vi "Init - Find Duplex.vi"(8 "error in (no error)":errorcluster, 11 "Compiled.Settings in":T1 {"Tx Packet Info"."targetPriority" min=1 step=1; "Tx Packet Info"."targetProcessor" min=-2 max=16 step=1; "Tx Packet Info"."Endianness" items=["big-endian"=0, "little-indian"=2]; "Rx Packet Info"."Endianness" items=["big-endian"=0, "little-indian"=2]}) -> (0 "error out":errorcluster, 3 "Compiled.Settings out":T1 {"Tx Packet Info"."targetPriority" min=1 step=1; "Tx Packet Info"."targetProcessor" min=-2 max=16 step=1; "Tx Packet Info"."Endianness" items=["big-endian"=0, "little-indian"=2]; "Rx Packet Info"."Endianness" items=["big-endian"=0, "little-indian"=2]})   [LabVIEW 2019, in "UDP-Custom-Device Engine.lvlib"]
uses:
  UDP-Custom-Device Engine.lvlib
  Shared/Compiled.Settings.ctl
  Shared/Types/Shared - Rx.PacketInfo.ctl
  Shared/Types/Shared - Channel Data Type.ctl
  Shared/Types/Shared - Buffered.PacketInfo.ctl
  Shared/Types/Shared - Pointer Encoding.ctl
  Shared/Types/Shared - Receive Buffer Options.ctl
  Shared/Types/Shared - Transmit Buffer Options.ctl
  Shared/Types/Shared - Duplex Settings.ctl
  Shared/Types/Shared - New Data Options.ctl
  Shared/Types/Shared - Thread Management.ctl
  Shared/Types/Shared - Tx.PacketInfo.ctl
  Shared/Types/Shared - Transmit Flag Options.ctl
  Shared/Types/Shared - Transmit Echo Options.ctl
  Shared/Types/Shared - Transmit Sim Options.ctl
  Shared/Types/Shared - Header Details.ctl
  Shared/Types/Shared - Custom Header.ctl
  Shared/UDP-Custom-Device Shared.lvlib
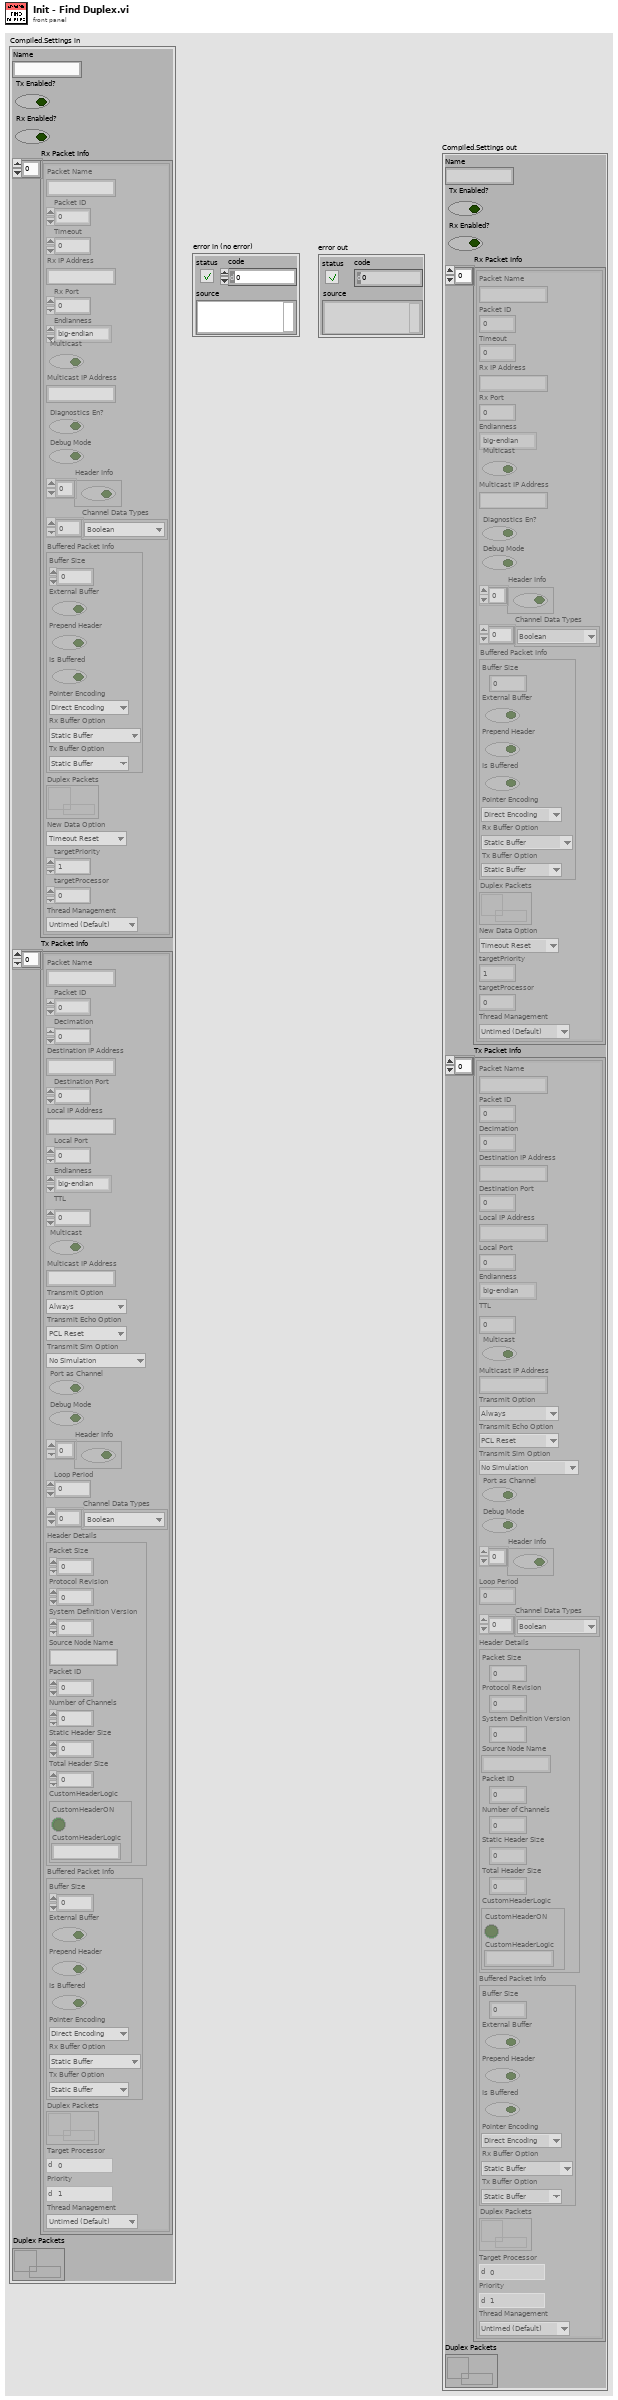
[diagram p1: front panel]
types:
  T1 = typedef "UDP-Custom-Device Shared.lvlib/Compiled.Settings.ctl" = cluster{"Name":string, "Tx Enabled?":bool, "Rx Enabled?":bool, "Rx Packet Info":T2[], "Tx Packet Info":T10[], "Duplex Packets":refnum<data-value>}
  T2 = typedef "UDP-Custom-Device Shared.lvlib/Shared - Rx.PacketInfo.ctl" = cluster{"Packet Name":string, "Packet ID":i32, "Timeout":i32, "Rx IP Address":string, "Rx Port":u16, "Endianness":u16, "Multicast":bool, "Multicast IP Address":string, "Diagnostics En?":bool, "Debug Mode":bool, "Header Info":bool[], "Channel Data Types":T3[], "Buffered Packet Info":T4, "Duplex Packets":refnum<data-value>, "New Data Option":T8, "targetPriority":i16, "targetProcessor":i8, "Thread Management":T9}
  T3 = typedef "UDP-Custom-Device Shared.lvlib/Shared - Channel Data Type.ctl" = enum16{"Boolean", "Single", "Double", "I8", "I16", "I32", "I64", "U8", "U16", "U32", "U64"}
  T4 = typedef "UDP-Custom-Device Shared.lvlib/Shared - Buffered.PacketInfo.ctl" = cluster{"Buffer Size":i32, "External Buffer":bool, "Prepend Header":bool, "Is Buffered":bool, "Pointer Encoding":T5, "Rx Buffer Option":T6, "Tx Buffer Option":T7}
  T5 = typedef "UDP-Custom-Device Shared.lvlib/Shared - Pointer Encoding.ctl" = enum16{"Direct Encoding", "Conversion Encoding"}
  T6 = typedef "UDP-Custom-Device Shared.lvlib/Shared - Receive Buffer Options.ctl" = enum16{"Static Buffer", "Circular Buffer", "Circular Buffer + Size", "Internal Cache", "Internal Cache + Size", "Ping Pong", "Ping Pong + Size"}
  T7 = typedef "UDP-Custom-Device Shared.lvlib/Shared - Transmit Buffer Options.ctl" = enum16{"Static Buffer", "FIFO Buffer", "FIFO Buffer + Port"}
  T8 = typedef "UDP-Custom-Device Shared.lvlib/Shared - New Data Options.ctl" = enum16{"Timeout Reset", "Counter"}
  T9 = typedef "UDP-Custom-Device Shared.lvlib/Shared - Thread Management.ctl" = enum16{"Untimed (Default)", "Timed (High Priority)"}
  T10 = typedef "UDP-Custom-Device Shared.lvlib/Shared - Tx.PacketInfo.ctl" = cluster{"Packet Name":string, "Packet ID":i32, "Decimation":u16, "Destination IP Address":string, "Destination Port":u16, "Local IP Address":string, "Local Port":u16, "Endianness":u16, "TTL":u16, "Multicast":bool, "Multicast IP Address":string, "Transmit Option":T11, "Transmit Echo Option":T12, "Transmit Sim Option":T13, "Port as Channel":bool, "Debug Mode":bool, "Header Info":bool[], "Loop Period":u32, "Channel Data Types":T3[], "Header Details":T14, "Buffered Packet Info":T4, "Duplex Packets":refnum<data-value>, "targetProcessor":i8, "targetPriority":i16, "Thread Management":T9}
  T11 = typedef "UDP-Custom-Device Shared.lvlib/Shared - Transmit Flag Options.ctl" = enum16{"Always", "One-Shot", "Toggle"}
  T12 = typedef "UDP-Custom-Device Shared.lvlib/Shared - Transmit Echo Options.ctl" = enum16{"PCL Reset", "Counter", "Mirror"}
  T13 = typedef "UDP-Custom-Device Shared.lvlib/Shared - Transmit Sim Options.ctl" = enum16{"No Simulation", "Counter", "Full Buffer", "FIFO Test", "FIFO + Port Test"}
  T14 = typedef "UDP-Custom-Device Shared.lvlib/Shared - Header Details.ctl" = cluster{"Packet Size":u16, "Protocol Revision":u8, "System Definition Version":u64, "Source Node Name":string, "Packet ID":u32, "Number of Channels":u32, "Static Header Size":u16, "Total Header Size":u16, "CustomHeaderLogic":T15}
  T15 = typedef "UDP-Custom-Device Shared.lvlib/Shared - Custom Header.ctl" = cluster{"CustomHeaderON":bool, "CustomHeaderLogic":string}
  T16 = typedef "UDP-Custom-Device Shared.lvlib/Shared - Duplex Settings.ctl" = cluster{"Transmit Packet ID":i32, "Receive Packet ID":i32, "Multicast":bool, "Multicast Address":string, "IP Address":string, "Port":u16, "TTL":u16, "Duplex Connection":refnum<k16>}
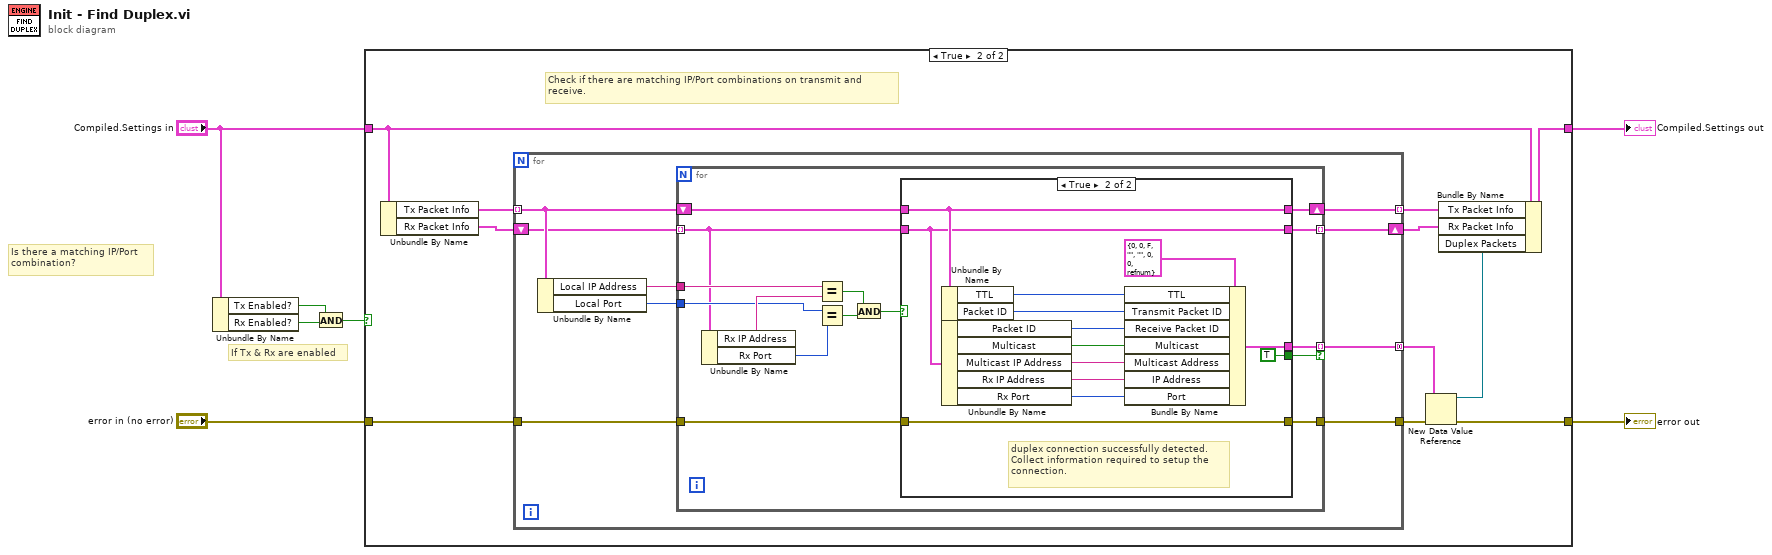
[diagram p0: block diagram]
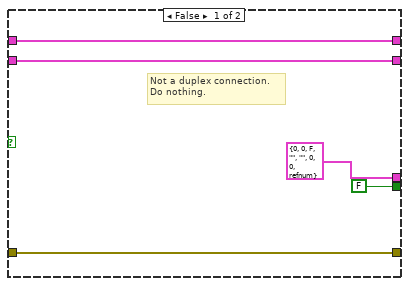
[diagram p3: hidden frame]
diagram:
  # "Is there a matching IP/Port\ncombination?"
  # "If Tx & Rx are enabled"
  n1 = Unbundle By Name("Compiled.Settings in") -> ("Tx Enabled?"=w4:bool, "Rx Enabled?"=w5:bool)
  n2 = And(x=w4, y=w5) -> (x .and. y?=w3:bool)
  n3 = case shown="True" w3 {
    tunnel: "error in (no error)" -> [w8 w20]
    tunnel: "Compiled.Settings in" -> [w9 w17]
    tunnel: [w9 w14] -> w2
    tunnel: [w8 w11] -> w1
    frame False {
      # "If both directions aren't enabled, we\nwill never have a duplicate IP address\nand port on a transmit and receive\npacket.\n\nWe will not have a duplex condition."
    }
    frame True {
      # "Check if there are matching IP/Port combinations on transmit and\nreceive."
      n4 = Unbundle By Name(w17) -> ("Tx Packet Info"=w18:T10[], "Rx Packet Info"=w19:T2[])
      n5 = for {
        tunnel: w20 -> [w27]
        tunnel: w18 -> [w26] mode=indexing
        shift-right: [w24] -> w15
        shift-left: w19 -> [w25]
        tunnel: [w23] -> w16 mode=indexing
        tunnel: [w22] -> w13 mode=concatenating
        tunnel: [w21] -> w12
        n6 = Unbundle By Name(w26) -> ("Local IP Address"=w29:string, "Local Port"=w28:u16)
        n7 = for {
          tunnel: w29 -> [w40]
          tunnel: w28 -> [w43]
          tunnel: w27 -> [w38]
          shift-right: [w36] -> w23
          shift-left: w26 -> [w35]
          tunnel: w25 -> [w33] mode=indexing
          tunnel: [w34] -> w24 mode=indexing
          tunnel: [w32] -> w22 mode=indexing if=w31
          tunnel: [w30] -> w21
          n8 = Unbundle By Name(w33) -> ("Rx IP Address"=w44:string, "Rx Port"=w39:u16)
          n9 = Equal?(x=w40, y=w44) -> (x = y?=w42:bool)
          n10 = Equal?(x=w43, y=w39) -> (x = y?=w41:bool)
          n11 = And(x=w42, y=w41) -> (x .and. y?=w37:bool)
          n12 = case shown="True" w37 {
            tunnel: w38 -> [w45 w51]
            tunnel: [w49 w62] -> w36
            tunnel: w35 -> [w49 w62]
            tunnel: [w48 w61] -> w34
            tunnel: w33 -> [w48 w61]
            tunnel: [T16 {"Transmit Packet ID"=0, "Receive Packet ID"=0, "Multicast"=FALSE, "Multicast Address"="", "IP Address"="", "Port"=0, "TTL"=0, "Duplex Connection"=refnum} ("Duplex Settings") w53] -> w32
            tunnel: [FALSE TRUE] -> w31
            tunnel: [w45 w51] -> w30
            frame False {
              # "Not a duplex connection.\nDo nothing."
            }
            frame True {
              # "duplex connection successfully detected.\nCollect information required to setup the\nconnection."
              n13 = Unbundle By Name(w62) -> ("TTL"=w50:u16, "Packet ID"=w59:i32)
              n14 = Unbundle By Name(w61) -> ("Packet ID"=w58:i32, "Multicast"=w57:bool, "Multicast IP Address"=w56:string, "Rx IP Address"=w55:string, "Rx Port"=w54:u16)
              n15 = Bundle By Name(cluster=T16 {"Transmit Packet ID"=0, "Receive Packet ID"=0, "Multicast"=FALSE, "Multicast Address"="", "IP Address"="", "Port"=0, "TTL"=0, "Duplex Connection"=refnum} ("Duplex Settings"), "TTL"=w50, "Transmit Packet ID"=w59, "Receive Packet ID"=w58, "Multicast"=w57, "Multicast Address"=w56, "IP Address"=w55, "Port"=w54) -> (w53:T16)
            }
          }
        }
      }
      n16 = New Data Value Reference(data value=w13, error in=w12) -> (data value reference=w10:refnum<data-value>, error out=w11:errorcluster)
      n17 = Bundle By Name(cluster=w17, "Tx Packet Info"=w16, "Rx Packet Info"=w15, "Duplex Packets"=w10) -> (w14:T1)
    }
  }
  "error out" <- w1
  "Compiled.Settings out" <- w2
